vi "PictureControl_MouseUp.vi"(7 "Finalize Movement":bool, 8 "error in":errorcluster, 10 "Coords":T5, 11 "Data in":T1={"Class"={"Ants"=refnum, "Layer"=refnum, "Templates"=refnum, "Icon"=refnum, "Glyph"=refnum, "Settings"=refnum, "Tools"=refnum, "History"=refnum}, "Ref"={"Add Layer"=refnum, "Remove Layer"=refnum, "Line Text"=[], "Body Text Spec"=refnum, "DNL_Font"=refnum, "glyph path str"=refnum, "templates path str"=refnum, "Arrow Up"=refnum, "Arrow Down"=refnum, "IE VI Ref"=refnum, "Glyphs tree"=refnum, "Templates tree"=refnum, "Layer Icon Text"=refnum, "Layer Template"=refnum, "Body Text"=refnum, "Search Templates"=refnum, "TextMarker"=refnum, "Tab Control"=refnum, "Search Glyphs"=refnum, "Line Color"=refnum, "DNL_Glyphs []"=refnum, "Fill Color"=refnum, "Tools"=refnum, "Icon"=refnum, "Preview"=refnum, "Ants"=refnum, "Terminals"=refnum, "menu reference"=refnum, "LayerNames"=[], "GlyphLoadAnimation"=refnum, "TemplateLoadAnimation"=refnum, "refreshGlyphs"=refnum, "refreshTemplates"=refnum}, "Support"={"AntsRect"={"left"=0, "top"=0, "right"=0, "bottom"=0}, "Mouse Move Coords"={"Horizontal"=0, "Vertical"=0}, "Mouse Down Coords"={"Horizontal"=0, "Vertical"=0}, "Temp Coord"={"Horizontal"=0, "Vertical"=0}, "Action"=enum."Default", "Edge Color"=4914962, "Fill Color"=16860, "Mouse Down?"=FALSE, "Draft Mode?"=FALSE, "Temp Icon"=bytes[3102], "CTRL Pressed"=FALSE, "Move Selection?"=FALSE, "AntsRect Orig"={"left"=0, "top"=0, "right"=0, "bottom"=0}, "Text"="", "TM Set?"=FALSE, "Mouse inside icon?"=FALSE, "Tool (old value)"=0, "Pencil Move Color"=0, "Swap Colors?"=FALSE, "Shift pressed?"=FALSE}}) -> (0 "error out":errorcluster, 3 "Data out":T1={"Class"={"Ants"=refnum, "Layer"=refnum, "Templates"=refnum, "Icon"=refnum, "Glyph"=refnum, "Settings"=refnum, "Tools"=refnum, "History"=refnum}, "Ref"={"Add Layer"=refnum, "Remove Layer"=refnum, "Line Text"=[], "Body Text Spec"=refnum, "DNL_Font"=refnum, "glyph path str"=refnum, "templates path str"=refnum, "Arrow Up"=refnum, "Arrow Down"=refnum, "IE VI Ref"=refnum, "Glyphs tree"=refnum, "Templates tree"=refnum, "Layer Icon Text"=refnum, "Layer Template"=refnum, "Body Text"=refnum, "Search Templates"=refnum, "TextMarker"=refnum, "Tab Control"=refnum, "Search Glyphs"=refnum, "Line Color"=refnum, "DNL_Glyphs []"=refnum, "Fill Color"=refnum, "Tools"=refnum, "Icon"=refnum, "Preview"=refnum, "Ants"=refnum, "Terminals"=refnum, "menu reference"=refnum, "LayerNames"=[], "GlyphLoadAnimation"=refnum, "TemplateLoadAnimation"=refnum, "refreshGlyphs"=refnum, "refreshTemplates"=refnum}, "Support"={"AntsRect"={"left"=0, "top"=0, "right"=0, "bottom"=0}, "Mouse Move Coords"={"Horizontal"=0, "Vertical"=0}, "Mouse Down Coords"={"Horizontal"=0, "Vertical"=0}, "Temp Coord"={"Horizontal"=0, "Vertical"=0}, "Action"=enum."Default", "Edge Color"=4914962, "Fill Color"=16860, "Mouse Down?"=FALSE, "Draft Mode?"=FALSE, "Temp Icon"=bytes[3102], "CTRL Pressed"=FALSE, "Move Selection?"=FALSE, "AntsRect Orig"={"left"=0, "top"=0, "right"=0, "bottom"=0}, "Text"="", "TM Set?"=FALSE, "Mouse inside icon?"=FALSE, "Tool (old value)"=0, "Pencil Move Color"=0, "Swap Colors?"=FALSE, "Shift pressed?"=FALSE}})   [LabVIEW 2020]
uses:
  Class/Ants/Ants.lvclass
  Class/FakedArray/FakedArray.lvclass
  vi.lib/LabVIEW Icon API/lv_icon/Classes/Icon/Icon.lvclass
  Class/Icon Library/Glyph.lvclass
  Class/Settings/Settings.lvclass
  Class/Tools/Tools Paint.lvclass
  History/History/History.lvclass
  Controls/SupportClass_Action.ctl
  <vilib>/Utility/miscctls.llb/LVPoint32TypeDef.ctl
  vi.lib/LabVIEW Icon API/lv_icon/Controls/IEColor.ctl
  Controls/Support Cluster.ctl
  lv_icon.lvlib
  Controls/References Cluster.ctl
  Controls/IE Classes.ctl
  Controls/Global Data.ctl
panel:
  out "Class.Icon":refnum<class "Icon.lvclass">
  out "Icon":refnum<class "Icon.lvclass">
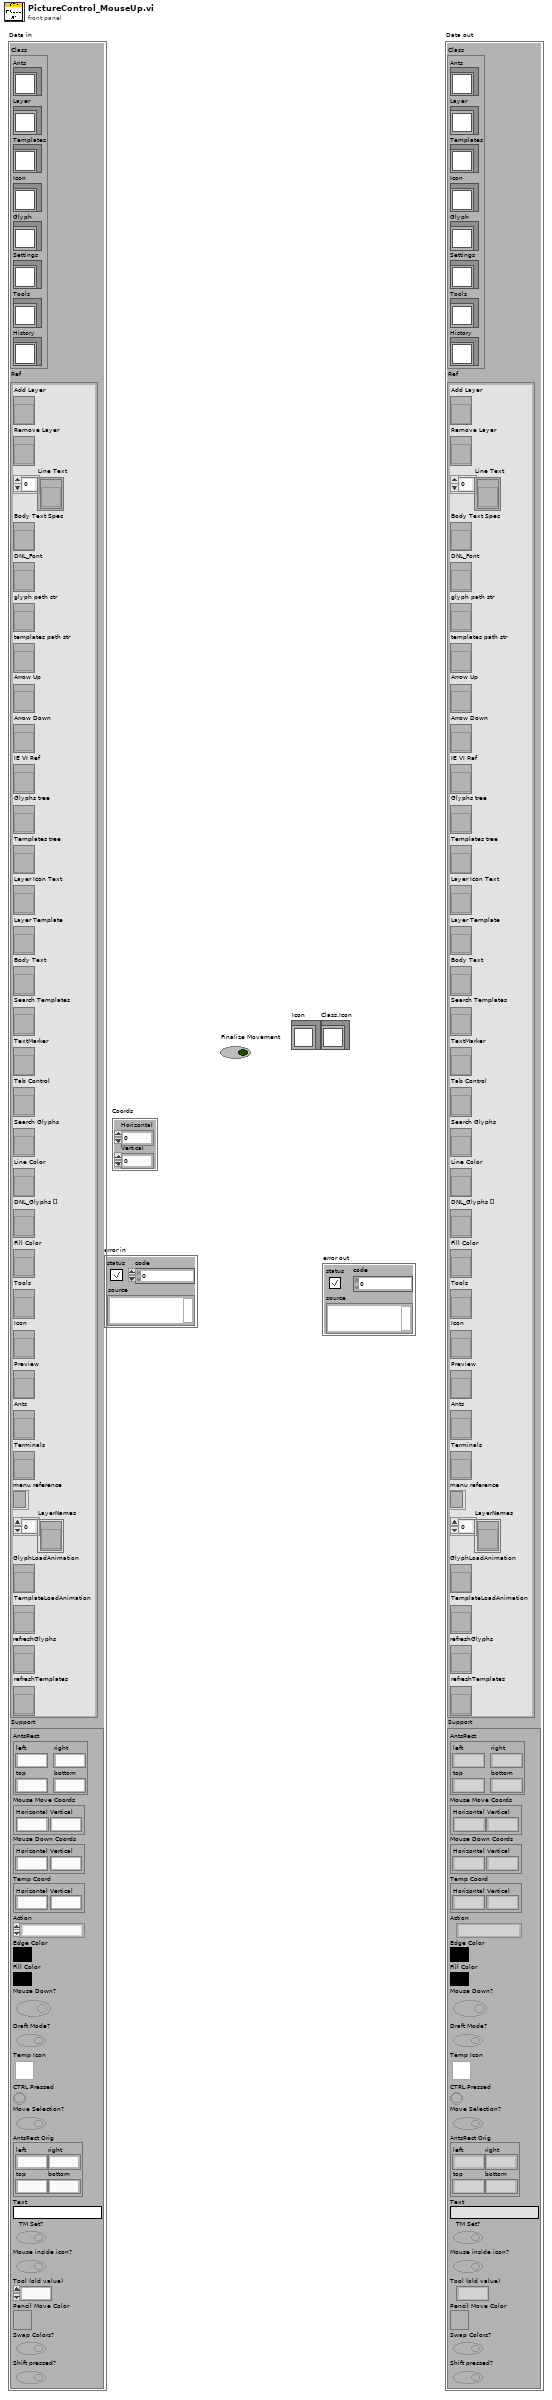
[diagram p1: front panel]
types:
  T1 = typedef "lv_icon.lvlib/Global Data.ctl" = cluster{"Class":T2, "Ref":T3, "Support":T4}
  T2 = typedef "lv_icon.lvlib/IE Classes.ctl" = cluster{"Ants":refnum<class "Ants.lvclass">, "Layer":refnum<class "FakedArray.lvclass">, "Templates":refnum<class "FakedArray.lvclass">, "Icon":refnum<class "Icon.lvclass">, "Glyph":refnum<class "Glyph.lvclass">, "Settings":refnum<class "Settings.lvclass">, "Tools":refnum<class "Tools Paint.lvclass">, "History":refnum<class "History.lvclass">}
  T3 = typedef "lv_icon.lvlib/References Cluster.ctl" = cluster{"Add Layer":refnum<vi>, "Remove Layer":refnum<vi>, "Line Text":refnum<vi>[], "Body Text Spec":refnum<vi>, "DNL_Font":refnum<vi>, "glyph path str":refnum<vi>, "templates path str":refnum<vi>, "Arrow Up":refnum<vi>, "Arrow Down":refnum<vi>, "IE VI Ref":refnum<vi>, "Glyphs tree":refnum<vi>, "Templates tree":refnum<vi>, "Layer Icon Text":refnum<vi>, "Layer Template":refnum<vi>, "Body Text":refnum<vi>, "Search Templates":refnum<vi>, "TextMarker":refnum<vi>, "Tab Control":refnum<vi>, "Search Glyphs":refnum<vi>, "Line Color":refnum<vi>, "DNL_Glyphs []":refnum<vi>, "Fill Color":refnum<vi>, "Tools":refnum<vi>, "Icon":refnum<vi>, "Preview":refnum<vi>, "Ants":refnum<vi>, "Terminals":refnum<vi>, "menu reference":refnum<k9>, "LayerNames":refnum<vi>[], "GlyphLoadAnimation":refnum<vi>, "TemplateLoadAnimation":refnum<vi>, "refreshGlyphs":refnum<vi>, "refreshTemplates":refnum<vi>}
  T4 = typedef "lv_icon.lvlib/Support Cluster.ctl" = cluster{"AntsRect":cluster{"left":i16, "top":i16, "right":i16, "bottom":i16}, "Mouse Move Coords":T5, "Mouse Down Coords":T5, "Temp Coord":T5, "Action":T6, "Edge Color":T7, "Fill Color":T7, "Mouse Down?":bool, "Draft Mode?":bool, "Temp Icon":picture, "CTRL Pressed":bool, "Move Selection?":bool, "AntsRect Orig":cluster{"left":i16, "top":i16, "right":i16, "bottom":i16}, "Text":string, "TM Set?":bool, "Mouse inside icon?":bool, "Tool (old value)":u32, "Pencil Move Color":u32, "Swap Colors?":bool, "Shift pressed?":bool}
  T5 = typedef "LVPoint32TypeDef.ctl" = cluster{"Horizontal":i32, "Vertical":i32}
  T6 = typedef "SupportClass_Action.ctl" = enum16{"Default", "Move Selection", "Glyph Library", "Tool"}
  T7 = typedef "IEColor.ctl" = u32
  T8 = cluster{"left":i16, "top":i16, "right":i16, "bottom":i16}
  T9 = cluster{"Horizontal":i32, "Vertical":i32, "Vertical 2":i32, "Vertical 3":i32}
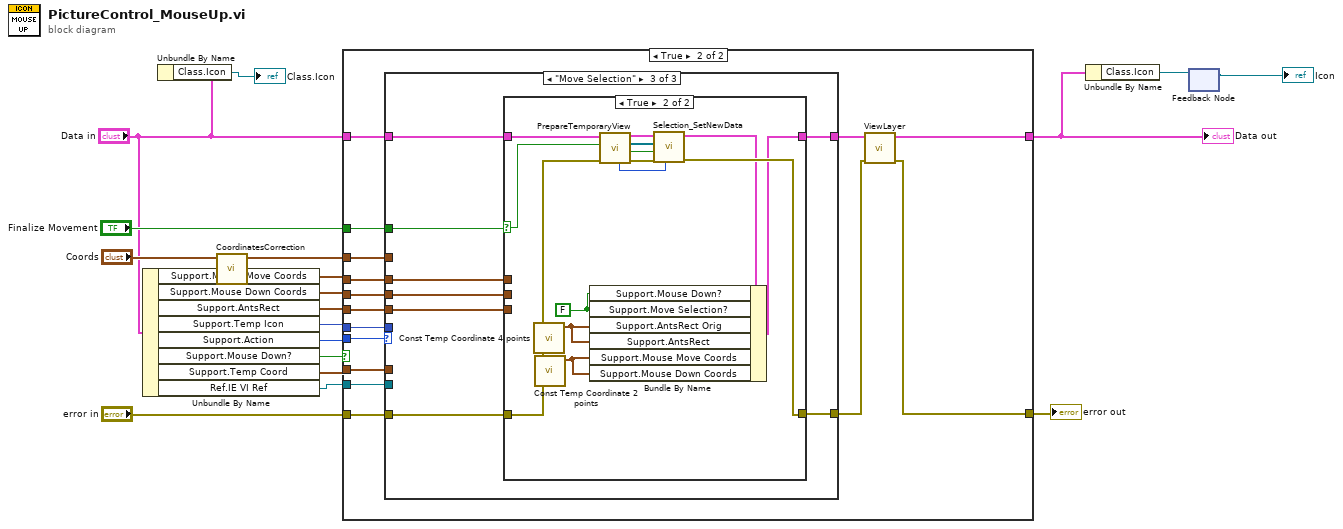
[diagram p0: block diagram]
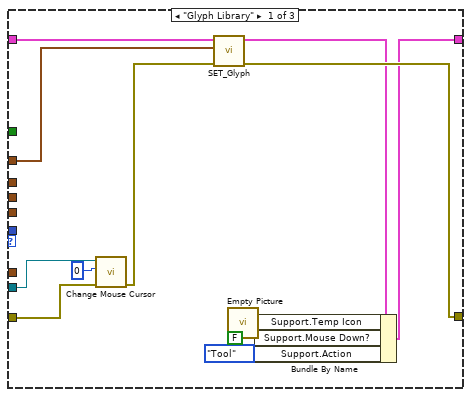
[diagram p3: hidden frame]
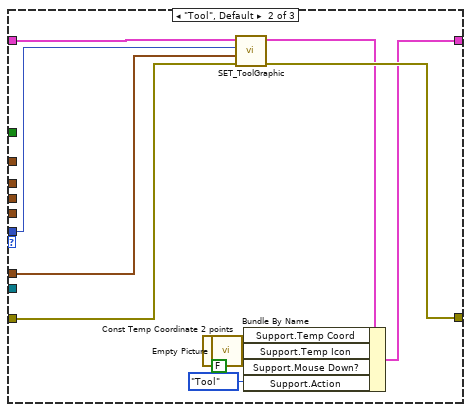
[diagram p4: hidden frame]
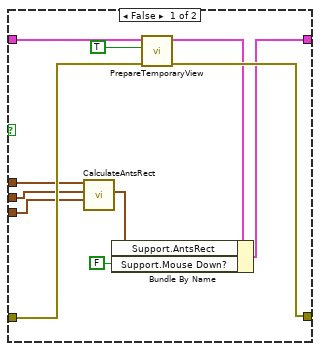
[diagram p5: hidden frame]
diagram:
  n1 = Unbundle By Name("Data in") -> ("Support.Mouse Move Coords"=w7:T5, "Support.Mouse Down Coords"=w8:T5, "Support.AntsRect"=w9:T8, "Support.Temp Icon"=w14:picture, "Support.Action"=w12:T6, "Support.Mouse Down?"=w13:bool, "Support.Temp Coord"=w16:T5, "Ref.IE VI Ref"=w6:refnum<vi>)
  n2 = Unbundle By Name("Data in") -> ("Class.Icon"=→"Class.Icon":refnum<class "Icon.lvclass">)
  n3 = call "CoordinatesCorrection.vi"("Coordinates In"="Coords") -> ("Corrected Out"=w15:T5)  [unwired: 10 out]
  n4 = case shown="True" w13 {
    tunnel: w12 -> [_ w32]
    tunnel: "error in" -> [w20 w35]
    tunnel: w14 -> [_ w31]
    tunnel: w15 -> [_ w30]
    tunnel: [w20 w33] -> w17
    tunnel: w16 -> [_ w29]
    tunnel: "Finalize Movement" -> [_ w28]
    tunnel: w9 -> [_ w27]
    tunnel: w8 -> [_ w26]
    tunnel: w7 -> [_ w25]
    tunnel: "Data in" -> [w19 w24]
    tunnel: [w19 w21] -> w4
    tunnel: w6 -> [_ w22]
    frame False {
    }
    frame True {
      n5 = case shown="\"Move Selection\"" w32 {
        tunnel: w35 -> [w46 w57 w66]
        tunnel: w31 -> [_ w52 _]
        tunnel: w30 -> [w44 _ _]
        tunnel: [w36 w54 w64] -> w23
        tunnel: [w47 w58 w65] -> w34
        tunnel: w29 -> [_ w51 _]
        tunnel: w28 -> [_ _ w63]
        tunnel: w27 -> [_ _ w60]
        tunnel: w26 -> [_ _ w61]
        tunnel: w25 -> [_ _ w62]
        tunnel: w24 -> [w40 w49 w59]
        tunnel: w22 -> [w38 _ _]
        frame "Glyph Library" {
          n6 = call "Change Mouse Cursor.vi"("error in (no error)"=w46, "icon"=u16 0, "VI reference (current VI)"=w38) -> ("error out"=w45:errorcluster)  [unwired: 8 out]
          n7 = call "SET_Glyph.vi"("error in"=w45, "Coordinates"=w44, "Data in"=w40) -> ("error out"=w47:errorcluster, "Data out"=w37:T1)  [unwired: 7 out]
          n8 = call "Empty Picture"() -> ("empty picture"=w41:picture)
          n9 = Bundle By Name(cluster=w37, "Support.Temp Icon"=w41, "Support.Mouse Down?"=FALSE ("Mouse Down?"), "Support.Action"=SupportClass_Action."Tool" ("Action")) -> (w36:T1)
        }
        frame "Tool", Default {
          n10 = call "Const Temp Coordinate 2 points.vi"() -> ("Const Temp Coordinate"=w50:T5)  [unwired: 11 out]
          n11 = call "Empty Picture"() -> ("empty picture"=w53:picture)
          n12 = call "SET_ToolGraphic.vi"("error in"=w57, "Temp Coord"=w51, "Temp Icon"=w52, "Data in"=w49) -> ("error out"=w58:errorcluster, "Data out"=w48:T1)  [unwired: 6 out]
          n13 = Bundle By Name(cluster=w48, "Support.Temp Coord"=w50, "Support.Temp Icon"=w53, "Support.Mouse Down?"=FALSE ("Mouse Down?"), "Support.Action"=SupportClass_Action."Tool" ("Action")) -> (w54:T1)
        }
        frame "Move Selection" {
          n14 = case shown="True" w63 {
            selector: w63 -> [_ w85]
            tunnel: w66 -> [w77 w90]
            tunnel: [w76 w89] -> w65
            tunnel: [w67 w84] -> w64
            tunnel: w62 -> [w74 _]
            tunnel: w61 -> [w73 _]
            tunnel: w60 -> [w72 _]
            tunnel: w59 -> [w69 w80]
            frame False {
              n15 = call "CalculateAntsRect.vi"("AntsRect"=w72, "Mouse Down Coords"=w73, "Mouse Move Coords"=w74) -> ("Rect"=w71:cluster{i32, i32, i32, i32})  [unwired: 8 out]
              n16 = call "PrepareTemporaryView.vi"("error in (no error)"=w77, "Valid Selection?"=TRUE, "Data in"=w69) -> ("error out"=w76:errorcluster, "Data out"=w68:T1)  [unwired: 2 in, 5 out]
              n17 = Bundle By Name(cluster=w68, "Support.AntsRect"=w71, "Support.Mouse Down?"=FALSE ("Mouse Down?")) -> (w67:T1)
            }
            frame True {
              w83 = FALSE ("Move Selection?")
              n18 = call "Const Temp Coordinate 4 points.vi"() -> ("Const Temp Coordinate"=w82:T9)  [unwired: 11 out]
              n19 = call "Const Temp Coordinate 2 points.vi"() -> ("Const Temp Coordinate"=w81:T5)  [unwired: 11 out]
              n20 = call "PrepareTemporaryView.vi"("error in (no error)"=w90, "Valid Selection?"=w85, "Data in"=w80) -> ("error out"=w91:errorcluster, "Highlighted?"=w87:bool, "All Layers out"=w88:refnum<class "Layer.lvclass">[], "Data out"=w79:T1, "#Active Layer"=w86:i32)  [unwired: 2 in, 2 out]
              n21 = call "Selection_SetNewData.vi"("#Active Layer"=w86, "error in"=w91, "Highlighted?"=w87, "All Layers In"=w88, "Data in"=w79) -> ("error out"=w89:errorcluster, "Data out"=w78:T1)  [unwired: 1 in, 3 out]
              n22 = Bundle By Name(cluster=w78, "Support.Mouse Down?"=w83, "Support.Move Selection?"=w83, "Support.AntsRect Orig"=w82, "Support.AntsRect"=w82, "Support.Mouse Move Coords"=w81, "Support.Mouse Down Coords"=w81) -> (w84:T1)
            }
          }
        }
      }
      n23 = call "ViewLayer.vi"("error in (no error)"=w34, "Data in"=w23) -> ("error out"=w33:errorcluster, "Data out"=w21:T1)  [unwired: 3 in, 5 out]
    }
  }
  "error out" <- w17
  "Data out" <- w4
  n24 = Unbundle By Name(w4) -> ("Class.Icon"=w3:refnum<class "Icon.lvclass">)
  n25 = feedback-in #1(w3) -> ()
  n26 = feedback #1() -> (→"Icon":refnum<class "Icon.lvclass">)  [unwired: 1 in]
